vi "MCL - Set Row Background Colour - Read.vi"(8 "Error In":errorcluster, 10 "Row index":i32, 11 "MCL":refnum<vi>) -> (0 "Error Out":errorcluster)   [LabVIEW 2016, in "Error Manager.lvlib" / "MCL.lvclass"]
doc: "Blank VI with error handling."
uses:
  MCL.lvclass
panel:
  # "Input\nInputs to the VI"
  # "Development\nControls or indicators that are useful for development or testing, but which are not outputs of the VI."
  # "Output\nOutputs of the VI"
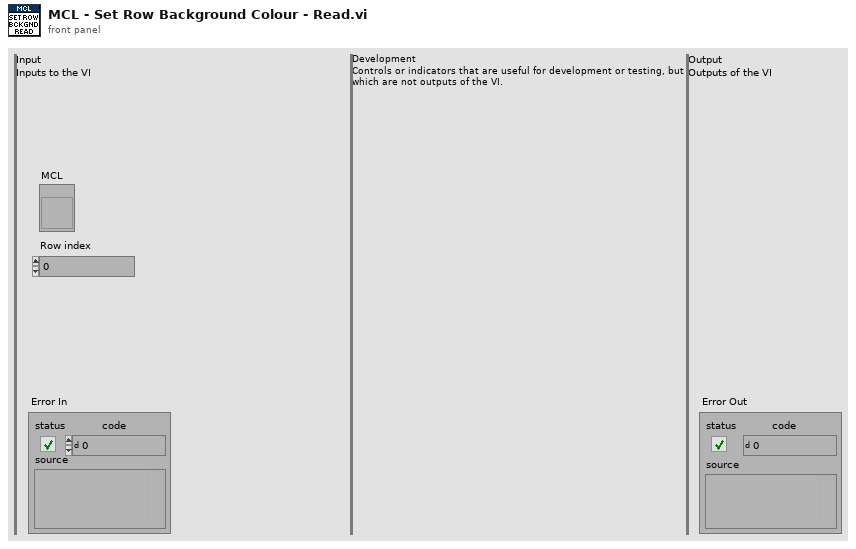
[diagram p1: front panel]
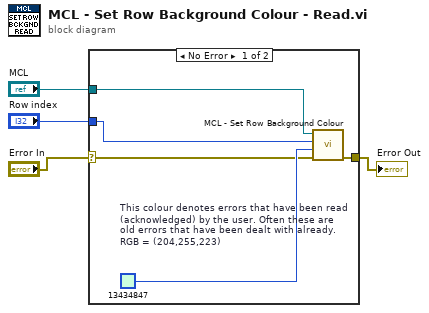
[diagram p0: block diagram]
diagram:
  n1 = case shown="No Error" "Error In" {
    selector: "Error In" -> [w8 w10]
    tunnel: [w7 w10] -> w3
    tunnel: "MCL" -> [w6 _]
    tunnel: "Row index" -> [w5 _]
    frame No Error {
      w9 = u32 13434847  # This colour denotes errors that have been read (acknowledged) by the user. Often these are old errors that have been dealt with already. RGB = (204,255,223)
      n2 = call "MCL - Set Row Background Colour.vi"("error in (no error)"=w8, "Row Background Colour"=w9, "Row index"=w5, "MCL Reference"=w6) -> ("error out"=w7:errorcluster)  [unwired: 7 in]
    }
    frame Error {
    }
  }
  "Error Out" <- w3
